vi "Destroy Data Channels.vi"(8 "error in":errorcluster, 11 "Node in":refnum<class "BLS Climate Chamber Template.lvclass">) -> (0 "error out":errorcluster, 3 "Node out":refnum<class "BLS Climate Chamber Template.lvclass">)   [LabVIEW 2023, in "BLS Climate Chamber Template.lvlib" / "BLS Climate Chamber Template.lvclass"]
uses:
  BLS Climate Chamber Template.lvclass
  BLS Climate Chamber Template.lvclass/BLS Climate Chamber Template.ctl
  <vilib>/Capabilities/Capabilities/High Level Capabilities/Climate Chamber/Climate Chamber.lvclass
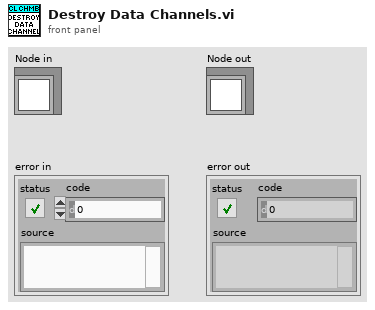
[diagram p1: front panel]
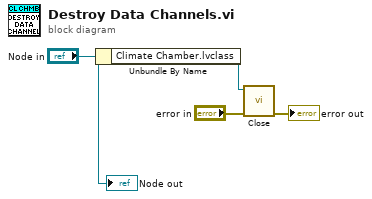
[diagram p0: block diagram]
diagram:
  n1 = Unbundle By Name("Node in") -> ("Climate Chamber.lvclass"=w4:refnum<class "Climate Chamber.lvclass">)
  n2 = call-dynamic "Close.vi"("error in"="error in", "Climate Chamber in"=w4) -> ("error out"=→"error out":errorcluster)  [unwired: 8 in, 1 out]
  "Node out" <- "Node in"
